vi "Handle Command.vi"(8 "error in (no error)":errorcluster, 10 "CMD in":refnum<class "Laser Enable CMD.lvclass">, 11 "Object In":refnum<class>) -> (0 "error out":errorcluster, 1 "Command Successful?":bool, 2 "CMD out":refnum<class "Laser Enable CMD.lvclass">, 3 "Object Out":refnum<class>)   [LabVIEW 2014, in "eCRDS Library.lvlib" / "Laser Enable CMD.lvclass"]
doc: "This VI will contain the code used to actually execute the request. If the request is successful, this will be indicated by the boolean output <b>Command Successful?</b>. The boolean output can then be used by the <b>Command Reply</b> which sends a reply if the reply queue is valid."
uses:
  Laser Enable CMD.lvclass
  Main/eCRDS.lvclass
  Laser Enable CMD.lvclass/Laser Enable CMD.ctl
  reusable/Instrument/Instrument.lvclass/Instrument.ctl
  <vilib>/DAQmx/write.llb/DAQmx Write (Digital 1D Bool NChan 1Samp 1Line).vi
  <vilib>/DAQmx/write.llb/DAQmx Write (Digital Bool 1Line 1Point).vi
  reusable/Instrument/Read Log Session.vi
  <vilib>/DAQmx/miscellaneous.llb/DAQmx Fill In Error Info.vi
  <userlib>/_Session Fwk/Session - Root.lvclass
  reusable/Session APIs/Session Log/System Log.lvclass
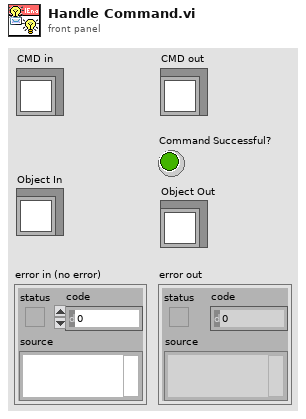
[diagram p1: front panel]
types:
  T1 = typedef "Session - Root.lvclass/Session Handle.ctl" = refnum<data-value>
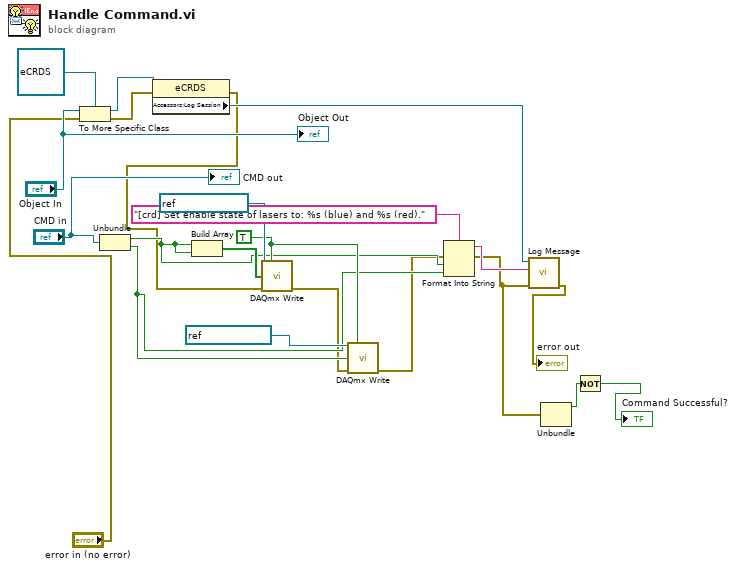
[diagram p0: block diagram]
diagram:
  w16 = TRUE ("auto start")
  n1 = To More Specific Class(target class=refnum<class "eCRDS.lvclass"> refnum ("eCRDS Library.lvlib:eCRDS"), reference="Object In", error in="error in (no error)") -> (specific class reference=w15:refnum<class "eCRDS.lvclass">, error out=w14:errorcluster)
  n2 = Unbundle("CMD in") -> (w12:bool, w11:bool)
  n3 = property class="eCRDS"(reference=w15, error in=w14) -> (error out=w5:errorcluster, "Accessors:Log Session"=w9:T1)  [unwired: 1 out]
  n4 = Build Array(w12, w12) -> (w19:bool[])
  n5 = call-poly <vilib>:"DAQmx Write.vi"("task/channels in"=refnum<k21> "Blue Enable", "auto start"=w16, "data"=w19, "error in"=w5) -> ("error out"=w8:errorcluster)  [unwired: 9 in, 2 out]
  n6 = call-poly <vilib>:"DAQmx Write.vi"("task/channels in"=refnum<k21> "Red Enable", "auto start"=w16, "data"=w11, "error in"=w8) -> ("error out"=w7:errorcluster)  [unwired: 9 in, 2 out]
  n7 = Format Into String(format string="[crd] Set enable state of lasers to: %s (blue) and %s (red).", error in=w7, w12, w11) -> (resulting string=w10:string, error out=w3:errorcluster)  [unwired: 1 in]
  n8 = call "Log Message.vi"("error in"=w3, "MSG In"=w10, "session in"=w9) -> ("error out"=→"error out":errorcluster)  [unwired: 7 in, 1 out]
  n9 = Unbundle(w3) -> ("status"=w2:bool)  [unwired: 2 out]
  n10 = Not(x=w2) -> (.not. x?=→"Command Successful?":bool)
  "CMD out" <- "CMD in"
  "Object Out" <- "Object In"
